vi "Initialize.vi"(7 "Serial Configuration":T1={"Baud Rate"=9600, "Parity"=0, "Data Bits"=8, "Stop Bits"=10, "Flow Control"=1} {"Flow Control" items=["None", "XON/XOFF", "RTS/CTS", "XON/XOFF & RTS/CTS", "DTR/DSR", "XON/XOFF & DTR/DSR"]; "Stop Bits" items=["1.0"=10, "1.5"=15, "2.0"=20]; "Data Bits" items=["7"=7, "8"=8]; "Parity" items=["None", "Odd", "Even", "Mark", "Space"]; "Baud Rate" items=["300"=300, "600"=600, "1200"=1200, "2400"=2400, "4800"=4800, "9600"=9600, "19200"=19200]}, 8 "error in (no error)":errorcluster, 11 "VISA resource name":refnum<visa-resource-name>) -> (0 "error out":errorcluster, 3 "VISA resource name out":refnum<visa-resource-name>)   [LabVIEW 2019, in "CAEN PSM.lvlib"]
doc: "Establishes communication with the instrument. Therefore, call this VI before calling other instrument driver VIs for this instrument. Generally, you need to call the Initialize VI only once at the beginning of an application."
uses:
  CAEN PSM.lvlib
panel:
  # "(c) 2012 CAEN SpA.  ALL RIGHTS RESERVED."
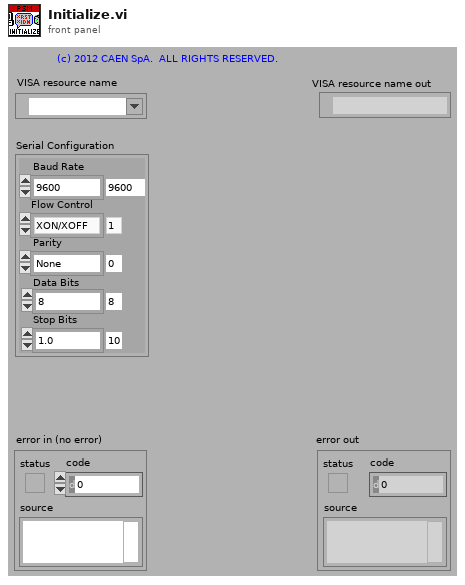
[diagram p1: front panel]
types:
  T1 = cluster{"Baud Rate":u32, "Parity":u16, "Data Bits":u16, "Stop Bits":u16, "Flow Control":u16}
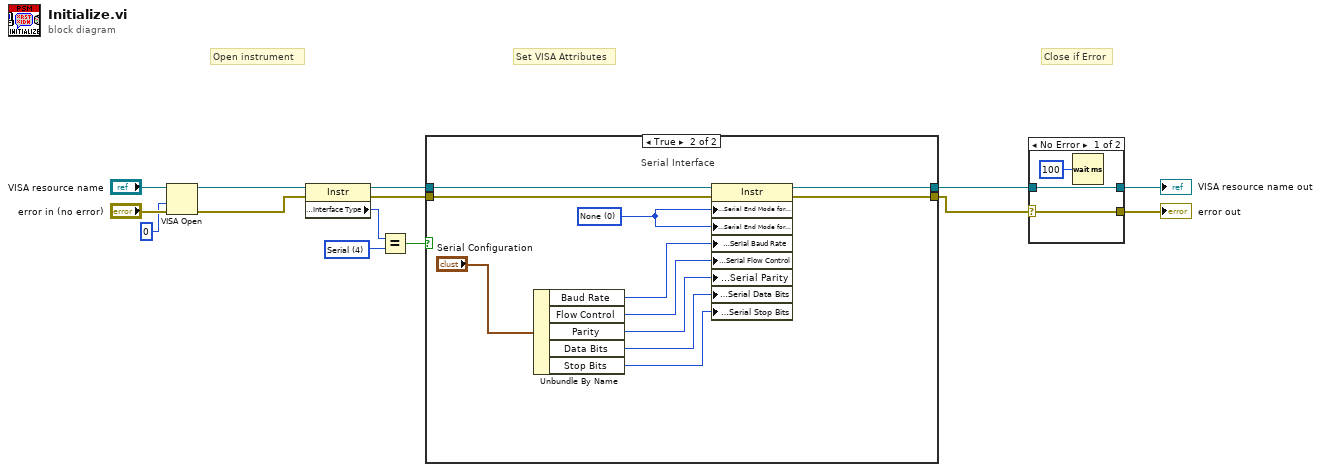
[diagram p0: block diagram]
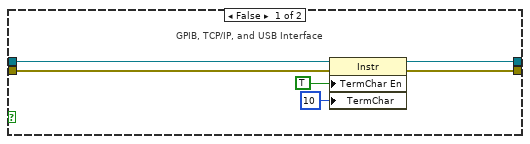
[diagram p2: hidden frame]
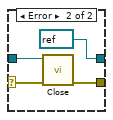
[diagram p3: hidden frame]
diagram:
  w8 = u16 4 items=["GPIB"=1, "VXI"=2, "GPIB-VXI"=3, "Serial"=4, "PXI"=5, "TCPIP"=6, "USB"=7] ("Interface Information:Interface Type")
  # "Set VISA Attributes"
  # "Close if Error"
  # "Open instrument"
  n1 = VISA Open(access mode=u32 0, error in (no error)="error in (no error)", VISA resource name="VISA resource name") -> (VISA resource name=w2:refnum<visa-resource-name>, error out=w1:errorcluster)  [unwired: 2 in]
  n2 = property class="Instr"(reference=w2, error in=w1) -> (reference out=w11:refnum<visa-resource-name>, error out=w10:errorcluster, "Interface Information:Interface Type"=w12:u16)
  n3 = Equal?(x=w12, y=w8) -> (x = y?=w9:bool)
  n4 = case shown="True" w9 {
    tunnel: [w17 w21] -> w4
    tunnel: [w18 w22] -> w3
    tunnel: w11 -> [w20 w30]
    tunnel: w10 -> [w19 w31]
    frame False {
      # "GPIB, TCP/IP, and USB Interface"
      n5 = property class="Instr"(reference=w20, error in=w19, "TermChar En"=TRUE ("Message Based Settings:Termination Character Enable"), "TermChar"=u8 10 ("Message Based Settings:Termination Character")) -> (reference out=w17:refnum<visa-resource-name>, error out=w18:errorcluster)
    }
    frame True {
      w29 = u16 0 items=["None", "LastBit", "TermChar"] ("Serial Settings:Serial End Mode for Reads")
      # "Serial Interface"
      n6 = Unbundle By Name("Serial Configuration") -> ("Baud Rate"=w28:u32, "Flow Control"=w24:u16, "Parity"=w26:u16, "Data Bits"=w27:u16, "Stop Bits"=w23:u16)
      n7 = property class="Instr"(reference=w30, error in=w31, "Serial Settings:Serial End Mode for Reads"=w29, "Serial Settings:Serial End Mode for Writes"=w29, "Serial Settings:Serial Baud Rate"=w28, "Serial Settings:Serial Flow Control"=w24, "Serial Settings:Serial Parity"=w26, "Serial Settings:Serial Data Bits"=w27, "Serial Settings:Serial Stop Bits"=w23) -> (reference out=w21:refnum<visa-resource-name>, error out=w22:errorcluster)
    }
  }
  n8 = case shown="No Error" w3 {
    selector: w3 -> [w33 w36]
    tunnel: w4 -> [w34 w37]
    tunnel: [w34 refnum<visa-resource-name> refnum ("VISA resource name out")] -> w6
    tunnel: [w33 w38] -> w5
    frame No Error {
      n9 = Wait (ms)(milliseconds to wait=u32 100) -> ()  [unwired: 1 out]
    }
    frame Error {
      n10 = call "Close.vi"("error in (no error)"=w36, "VISA resource name"=w37) -> ("error out"=w38:errorcluster)  [unwired: 9 in]
    }
  }
  "VISA resource name out" <- w6
  "error out" <- w5
